vi "Simple TCP - Client - modified for VIRES.vi"() -> ()   [LabVIEW 2018]
doc: "Demonstrates how to open a connection to an TCP server, read the data being sent, and display the data on a chart. This VI is designed to stop if the TCP connection is terminated."
uses:
  SCP.lvlib
panel:
  in  "New Scenario":string
  in  "Step Size (1 step = 17 ms)":i16
  in  "Simulation Time (s)":i16
  in  "Server Closed 2":string="The server VI closed the connection."
  out "data 2":string
  in  "Selection":T1(ring)
  in  "Command":string="<SimCtrl><Stop /></SimCtrl>\n<SimCtrl><Project name=\"SampleProject\" path=\"/home/philip/Vires21/VTD.2.1/Data/Projects/SampleProject\" /></SimCtrl>\n<SimCtrl><LoadScenario filename=\"/home/philip/Vires21/VTD.2.1/Data/Projects/SampleProject/Scenarios/traffic_demo.xml\" /><Start mode=\"operation\" /></SimCtrl>"
  in  "Write":bool
  in  "Server Closed":string="The server VI closed the connection."
  in  "Stop":bool
  # "Overview: Demonstrates the use of the TCP functions to connect to a TCP server VI and receive data.\nInstructions:\n1. Ensure Simple TCP - Server.vi is already running.\n2. Run the VI.\n3. Click Stop to stop the VI. Note that if you stop the server VI, this VI will stop automatically."
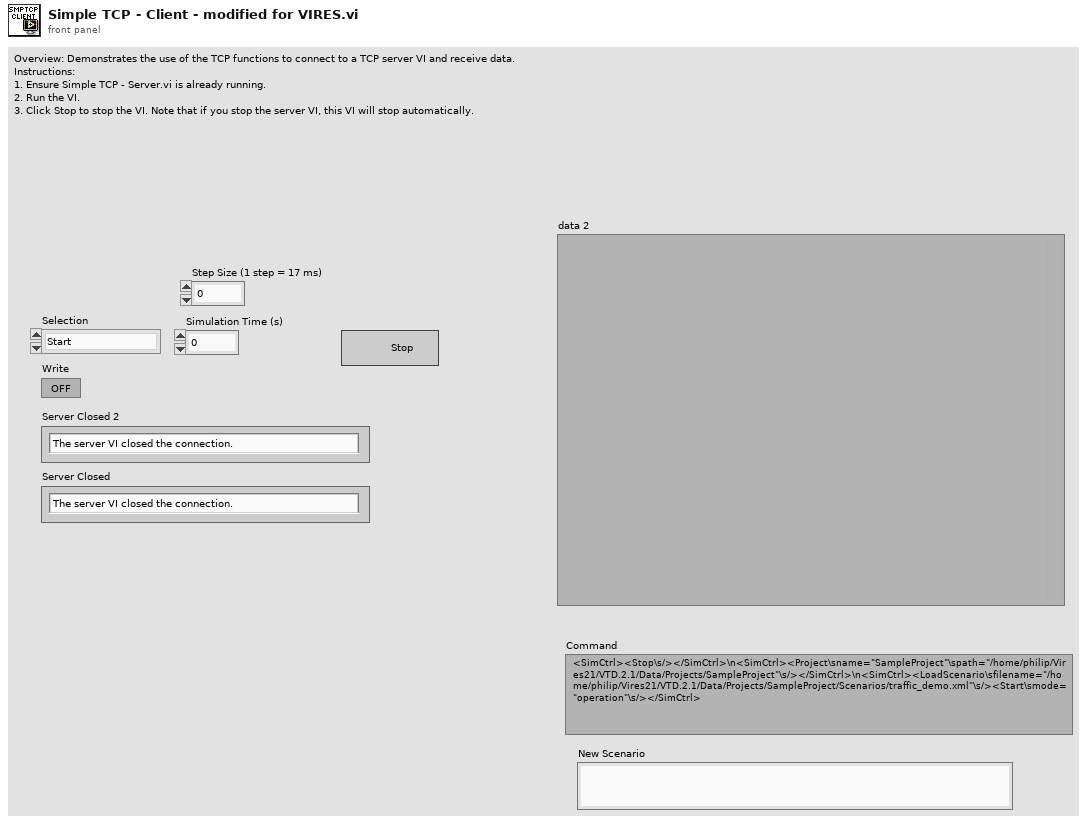
[diagram p1: front panel]
types:
  T1 = enum16{"Start", "Stop", "Pause", "Restart", "Step", "Change Scenario"}
  T2 = enum16{"Standard", "Buffered", "CRLF", "Immediate"}
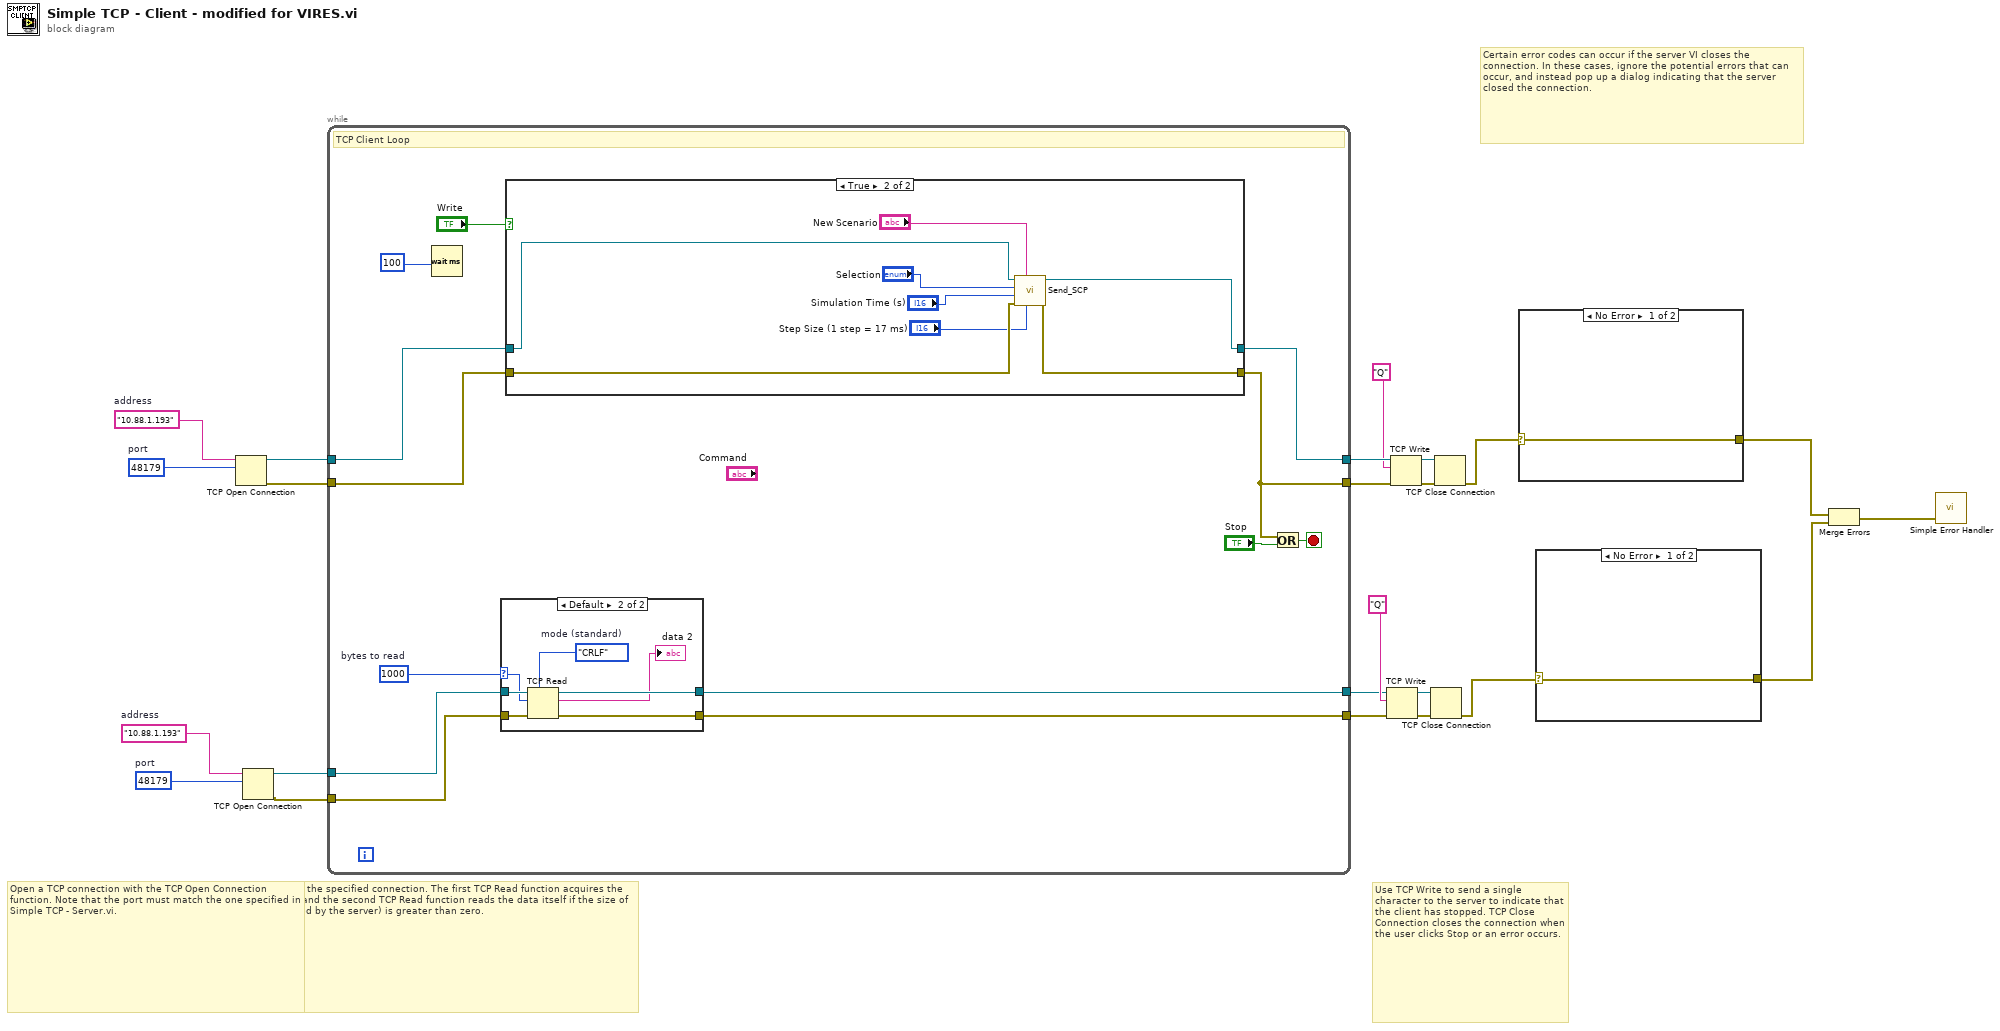
[diagram p0: block diagram]
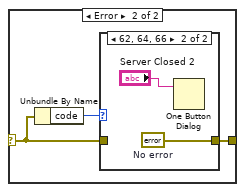
[diagram p4: hidden frame]
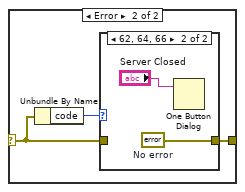
[diagram p6: hidden frame]
diagram:
  w13 = u16 48179  # port
  w12 = "10.88.1.193"  # address
  w16 = u16 48179  # port
  w17 = "10.88.1.193"  # address
  # "Certain error codes can occur if the server VI closes the connection. In these cases, ignore the potential errors that can occur, and instead pop up a dialog indicating that the server closed the connection."
  # "Use TCP Write to send a single character to the server to indicate that the client has stopped. TCP Close Connection closes the connection when the user clicks Stop or an error occurs."
  # "Read the data on the specified connection. The first TCP Read function acquires the size of the data, and the second TCP Read function reads the data itself if the size of the data (specified by the server) is greater than zero."
  # "Open a TCP connection with the TCP Open Connection function. Note that the port must match the one specified in Simple TCP - Server.vi."
  n1 = TCP Open Connection(address=w17, remote port or service name=w16) -> (connection ID=w15:refnum<k5>, error out=w14:errorcluster)  [unwired: 3 in]
  n2 = TCP Open Connection(address=w12, remote port or service name=w13) -> (connection ID=w11:refnum<k5>, error out=w10:errorcluster)  [unwired: 3 in]
  n3 = while {
    tunnel: w14 -> [w32]
    tunnel: w15 -> [w30]
    tunnel: [w33] -> w22
    tunnel: [w34] -> w20
    tunnel: w11 -> [w27]
    tunnel: w10 -> [w28]
    tunnel: [w26] -> w5
    tunnel: [w25] -> w4
    stop <- w35 stop-if-true
    w24 = 1000  # bytes to read
    # "TCP Client Loop"
    n4 = Wait (ms)(milliseconds to wait=u32 100) -> ()  [unwired: 1 out]
    n5 = case shown="Default" w24 {
      selector: w24 -> [_ w41]
      tunnel: w27 -> [w38 w45]
      tunnel: w28 -> [w37 w44]
      tunnel: [w38 w43] -> w26
      tunnel: [w37 w42] -> w25
      frame ..0 {
        # "The server has not written any data"
      }
      frame Default {
        w39 = T2."CRLF"  # mode (standard)
        n6 = TCP Read(connection ID=w45, bytes to read=w41, error in (no error)=w44, 7:w39) -> (connection ID out=w43:refnum<k5>, data out=→"data 2":string, error out=w42:errorcluster)  [unwired: 1 in]
      }
    }
    n7 = case shown="True" "Write" {
      tunnel: [w46 w55] -> w34
      tunnel: [w47 w54] -> w33
      tunnel: w30 -> [w47 w52]
      tunnel: w32 -> [w46 w53]
      frame False {
      }
      frame True {
        n8 = call "Send_SCP.vi"("Step Size (1 step = 17 ms)"="Step Size (1 step = 17 ms)", "New Scenario"="New Scenario", "error in (no error)"=w53, "Simulation Time (s)"="Simulation Time (s)", "Selection"="Selection", "TCP Network Connection in"=w52) -> ("error out"=w55:errorcluster, "TCP Network Connection out"=w54:refnum<k5>)  [unwired: 4 in]
      }
    }
    n9 = Or(x=w34, y="Stop") -> (x .or. y?=w35:bool)
  }
  n10 = TCP Write(connection ID=w5, data in="Q", error in (no error)=w4) -> (connection ID out=w6:refnum<k5>, error out=w7:errorcluster)  [unwired: 2 out]
  n11 = TCP Write(connection ID=w22, data in="Q", error in (no error)=w20) -> (connection ID out=w23:refnum<k5>, error out=w21:errorcluster)  [unwired: 2 out]
  n12 = TCP Close Connection(connection ID=w6, error in (no error)=w7) -> (error out=w9:errorcluster)  [unwired: 1 in, 1 out]
  n13 = TCP Close Connection(connection ID=w23, error in (no error)=w21) -> (error out=w18:errorcluster)  [unwired: 1 in, 1 out]
  n14 = case shown="No Error" w18 {
    selector: w18 -> [w56 w58]
    tunnel: [w56 w57] -> w2
    frame No Error {
    }
    frame Error {
      n15 = Unbundle By Name(w58) -> ("code"=w59:i32)
      n16 = case shown="62, 64, 66" w59 {
        tunnel: w58 -> [w60 _]
        tunnel: [w60 w62] -> w57
        frame Default {
        }
        frame 62, 64, 66 {
          w62 = errorcluster {"status"=FALSE, "code"=0, "source"=""}  # No error
          n17 = One Button Dialog(message="Server Closed") -> ()  [unwired: 1 in, 1 out]
        }
      }
    }
  }
  n18 = case shown="No Error" w9 {
    selector: w9 -> [w63 w65]
    tunnel: [w63 w64] -> w3
    frame No Error {
    }
    frame Error {
      n19 = Unbundle By Name(w65) -> ("code"=w66:i32)
      n20 = case shown="62, 64, 66" w66 {
        tunnel: w65 -> [w67 _]
        tunnel: [w67 w69] -> w64
        frame Default {
        }
        frame 62, 64, 66 {
          w69 = errorcluster {"status"=FALSE, "code"=0, "source"=""}  # No error
          n21 = One Button Dialog(message="Server Closed 2") -> ()  [unwired: 1 in, 1 out]
        }
      }
    }
  }
  n22 = Merge Errors(w2, w3) -> (w1:errorcluster)
  n23 = call <vilib>:"Simple Error Handler.vi"("error in (no error)"=w1) -> ()  [unwired: 4 in, 5 out]
